vi "Get Topic Attributes.vi"(8 "error in (no error)":errorcluster, 11 "Topic in":refnum<class "Topic.lvclass">) -> (0 "error out":errorcluster, 2 "Topic Attributes":T1[](array[typedef]), 3 "Topic out":refnum<class "Topic.lvclass">)   [LabVIEW 2015, in "NI_AWS_SNS.lvlib" / "Topic.lvclass"]
doc: "Returns all of the properties of a topic. Topic properties returned might differ based on the authorization of the user."
uses:
  Topic.lvclass
  Topic Attribute Value Pair.ctl
  Topic Attribute.ctl
  Core/HTTP Request/Name Value Pair.ctl
  Core/HTTP Request/Request Options.ctl
  Core/HTTP Request/Region handling.ctl
  Core/HTTP Request/URL formatting.ctl
  Core/ARN/ARN.lvclass/ARN.ctl
  Core/ARN/Read ARN.vi
  Core/HTTP Request/HTTP Request.lvclass
  XML Parsing/NI_XML Parsing.lvlib
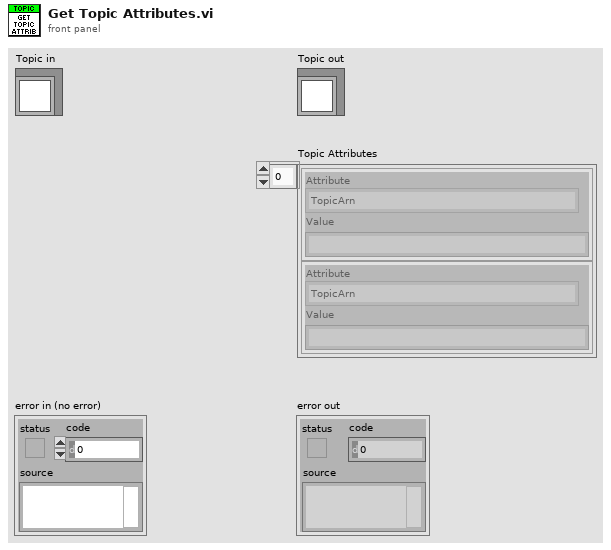
[diagram p1: front panel]
types:
  T1 = typedef "NI_AWS_SNS.lvlib/Topic.lvclass/Topic Attribute Value Pair.ctl" = cluster{"Attribute":T2, "Value":string}
  T2 = typedef "NI_AWS_SNS.lvlib/Topic.lvclass/Topic Attribute.ctl" = enum16{"TopicArn", "Owner", "Policy", "DisplayName", "SubscriptionsPending", "SubscriptionsConfirmed", "SubscriptionsDeleted", "DeliveryPolicy", "EffectiveDeliveryPolicy"}
  T3 = typedef "NI_AWS_Core.lvlib/HTTP Request.lvclass/Request Options.ctl" = cluster{"request headers":T4[], "request parameters":T4[], "request body":string, "region handling":T5, "URL formatting":T6}
  T4 = typedef "NI_AWS_Core.lvlib/HTTP Request.lvclass/Name Value Pair.ctl" = cluster{"name":string, "value":string}
  T5 = typedef "NI_AWS_Core.lvlib/HTTP Request.lvclass/Region handling.ctl" = enum16{"use region everywhere", "use region (authentication only)", "use region (URL only)", "ignore region everwhere"}
  T6 = typedef "NI_AWS_Core.lvlib/HTTP Request.lvclass/URL formatting.ctl" = enum16{"region-", "region."}
  T7 = typedef "NI_AWS_Core.lvlib/HTTP Request.lvclass/Response.ctl" = cluster{"Headers":string, "Body":string}
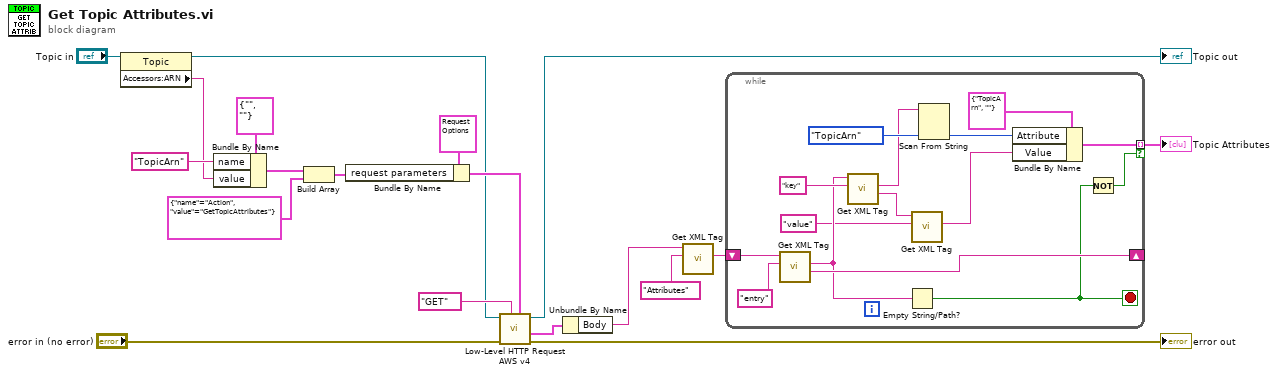
[diagram p0: block diagram]
diagram:
  n1 = property class="Topic"(reference="Topic in") -> (reference out=w2:refnum<class "Topic.lvclass">, "Accessors:ARN"=w17:string)  [unwired: 1 in, 1 out]
  n2 = Bundle By Name(cluster=T4 {"name"="", "value"=""} ("element"), "name"="TopicArn", "value"=w17) -> (w12:T4)
  n3 = Build Array(w12, T4 {"name"="Action", "value"="GetTopicAttributes"} ("Cluster")) -> (w10:T4[])
  n4 = Bundle By Name(cluster=T3 {"request headers"=[], "request parameters"=[{"name"="Action", "value"="ListQueues"}], "request body"="", "region handling"=enum."use region everywhere", "URL formatting"=enum."region."} ("Request Options"), "request parameters"=w10) -> (w3:T3)
  n5 = call "Low-Level HTTP Request AWS v4.vi"("Request Options"=w3, "HTTP-Verb"="GET", "error in (no error)"="error in (no error)", "AWS Core in"=w2) -> ("error out"=→"error out":errorcluster, "Response"=w5:T7, "AWS Core out"=→"Topic out":refnum<class "Topic.lvclass">)  [unwired: 4 in, 1 out]
  n6 = Unbundle By Name(w5) -> ("Body"=w9:string)
  n7 = call "Get XML Tag.vi"("Tag name"="Attributes", "XML String in"=w9) -> ("Tag value"=w7:string)  [unwired: 5 in, 4 out]
  n8 = while {
    shift-right: [w33] -> _
    shift-left: w7 -> [w34]
    tunnel: [w25] -> w6 mode=indexing if=w20
    stop <- w21 stop-if-true
    n9 = call "Get XML Tag.vi"("Tag name"="entry", "XML String in"=w34) -> ("Remaining string"=w33:string, "Tag value"=w30:string)  [unwired: 5 in, 3 out]
    n10 = call "Get XML Tag.vi"("Tag name"="key", "XML String in"=w30) -> ("Remaining string"=w29:string, "Tag value"=w23:string)  [unwired: 5 in, 3 out]
    n11 = Empty String/Path?(string/path=w30) -> (empty?=w21:bool)
    n12 = call "Get XML Tag.vi"("Tag name"="value", "XML String in"=w29) -> ("Tag value"=w26:string)  [unwired: 5 in, 4 out]
    n13 = Scan From String(input string=w23, default 1=Topic_Attribute."TopicArn" ("Attribute")) -> (output 1=w22:T2)  [unwired: 3 in, 3 out]
    n14 = Bundle By Name(cluster=T1 {"Attribute"=enum."TopicArn", "Value"=""} ("Attribute Value Pair"), "Attribute"=w22, "Value"=w26) -> (w25:T1)
    n15 = Not(x=w21) -> (.not. x?=w20:bool)
  }
  "Topic Attributes" <- w6
